vi "sweep_setup.vi"(8 "error in (no error)":errorcluster, 10 "Check scan settings":T1={"Start voltage (V)"=0.0, "End voltage (V)"=0.0, "Number of steps"=0, "Settling delay (ms)"=0.0, "Dual sweep"=0, "Stabilisation time (s)"=0.0, "Stabilisation mode"=0, "Stabilisation value (V or A) "=0.0, "No. of repeat scans"=0.0, "Repeat scans"=0, "Logarithmic sweep"=0, "Electrode configuration"=0, "Sweep mode"=0, "Auto settling delay"=1, "Pulse off time (ms)"=0.0, "Integration time (ms)"=1.0, "Current range"=0, "Enable display"=0, "Enable concurrent measurements"=1, "Concurrent measurements"=1} {"Concurrent measurements" items=["Volts", "Current", "Resistance", "Volt, Current", "Volts, Resistance", "Current, Resistance", "All"]; "Enable concurrent measurements" items=["False", "True"]; "Enable display" items=["False", "True"]; "Current range" items=["Auto", "1 uA", "10 uA", "100 uA", "1 mA", "10 mA", "100 mA", "1 A"]; "Integration time (ms)" min=0.2 max=200.0; "Pulse off time (ms)" min=0.0; "Auto settling delay" items=["False", "True"]; "Sweep mode" items=["Staircase", "Pulsed"]; "Electrode configuration" items=["2-wire", "4-wire"]; "Logarithmic sweep" items=["False", "True"]; "Repeat scans" items=["False", "True"]; "No. of repeat scans" min=1.0 step=1.0; "Stabilisation mode" items=["V", "I"]; "Dual sweep" items=["False", "True"]; "Settling delay (ms)" min=0.0 max=999999.9}, 11 "VISA Refnum in":refnum<visa-resource-name>) -> (0 "error out":errorcluster, 2 "Voltage list":dbl[](array[numeric]), 3 "VISA Refnum out":refnum<visa-resource-name>)   [LabVIEW 2016]
uses:
  TypeDefs/settings.ctl
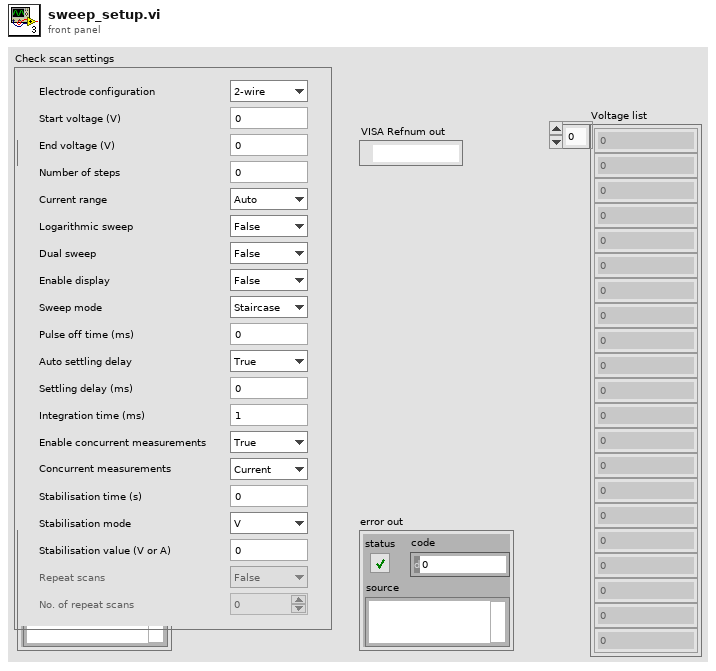
[diagram p1: front panel]
types:
  T1 = typedef "settings.ctl" = cluster{"Start voltage (V)":dbl, "End voltage (V)":dbl, "Number of steps":u32, "Settling delay (ms)":dbl, "Dual sweep":u16, "Stabilisation time (s)":dbl, "Stabilisation mode":u16, "Stabilisation value (V or A) ":dbl, "No. of repeat scans":dbl, "Repeat scans":u16, "Logarithmic sweep":u16, "Electrode configuration":u16, "Sweep mode":u16, "Auto settling delay":u16, "Pulse off time (ms)":dbl, "Integration time (ms)":dbl, "Current range":u16, "Enable display":u16, "Enable concurrent measurements":u16, "Concurrent measurements":u16}
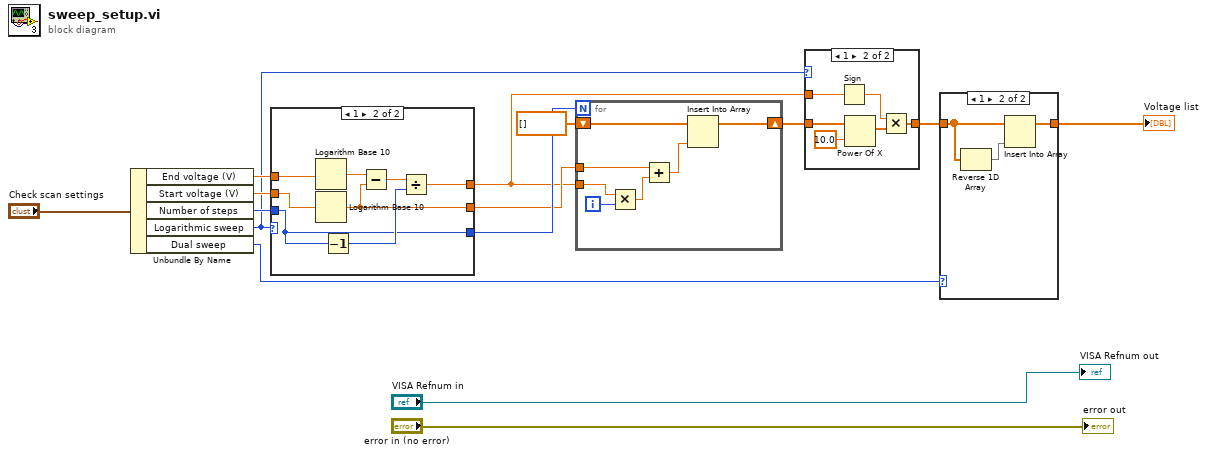
[diagram p0: block diagram]
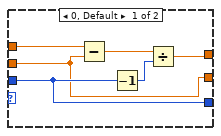
[diagram p3: hidden frame]
diagram:
  n1 = Unbundle By Name("Check scan settings") -> ("End voltage (V)"=w12:dbl, "Start voltage (V)"=w13:dbl, "Number of steps"=w11:u32, "Logarithmic sweep"=w7:u16, "Dual sweep"=w8:u16)
  n2 = case shown="1" w7 {
    tunnel: w13 -> [w17 w22]
    tunnel: w12 -> [w21 w23]
    tunnel: w11 -> [w18 w25]
    tunnel: [w19 w26] -> w3
    tunnel: [w18 w25] -> w10
    tunnel: [w17 w24] -> w9
    frame 0, Default {
      n3 = Subtract(x=w21, y=w17) -> (x-y=w16:dbl)
      n4 = Decrement(x=w18) -> (x-1=w20:u32)
      n5 = Divide(x=w16, y=w20) -> (x/y=w19:dbl)
    }
    frame 1 {
      n6 = Logarithm Base 10(1:w23) -> (0:w28:dbl)
      n7 = Logarithm Base 10(1:w22) -> (0:w24:dbl)
      n8 = Decrement(x=w25) -> (x-1=w29:u32)
      n9 = Subtract(x=w28, y=w24) -> (x-y=w27:dbl)
      n10 = Divide(x=w27, y=w29) -> (x/y=w26:dbl)
    }
  }
  n11 = for {
    N: w10 -> [_]
    shift-right: [w35] -> w6
    shift-left: dbl[] [] -> [w36]
    tunnel: w3 -> [w32]
    tunnel: w9 -> [w33]
    i -> [w31]
    n12 = Multiply(x=w32, y=w31) -> (x*y=w34:dbl)
    n13 = Add(x=w33, y=w34) -> (x+y=w30:dbl)
    n14 = Insert Into Array(array=w36, new element=w30) -> (w35:dbl[])  [unwired: 1 in]
  }
  n15 = case shown="1" w7 {
    tunnel: w6 -> [w37 w42]
    tunnel: [w37 w40] -> w5
    tunnel: w3 -> [_ w38]
    frame 0, Default {
    }
    frame 1 {
      n16 = Sign(1:w38) -> (0:w39:dbl)
      n17 = Power Of X(1:10.0 ("y"), 2:w42) -> (0:w41:dbl[])
      n18 = Multiply(x=w39, y=w41) -> (x*y=w40:dbl[])
    }
  }
  n19 = case shown="1" w8 {
    tunnel: w5 -> [w44 w47]
    tunnel: [w44 w45] -> w15
    frame 0, Default {
    }
    frame 1 {
      n20 = Reverse 1D Array(array=w47) -> (reversed array=w46:dbl[])
      n21 = Insert Into Array(array=w47, new element=w46) -> (w45:dbl[])  [unwired: 1 in]
    }
  }
  "Voltage list" <- w15
  "error out" <- "error in (no error)"
  "VISA Refnum out" <- "VISA Refnum in"
